vi "ATF - Datalog Redundant.vi"() -> ()   [LabVIEW 2022 SP3]
doc: "Datalog and display software modified"
uses:
  Source Code/Control/SeCrTs-Enum.ctl
  Source Code/Globals/SeCrTS-DD globals.vi
panel:
  out "Backlog Storage":i32
  out "Backlog Pump":i32
  out "Logging Mode":string
  out "cmd":bool=TRUE
  out "Storage Connected?":bool
  in  "Pump IP Address":string="169.254.31.109"
  in  "Storage IP Address":string="169.254.19.218"
  out "Datalog Title":string
  in  "Exit":bool
  out "Log Period(Min)":dbl
  out "Logging?":bool
  out "Pumb Connected?":bool
  out "error Out":errorcluster
  # "ATF PUMP AND STORAGE"
  # "DATALOG  REDUNDANT"
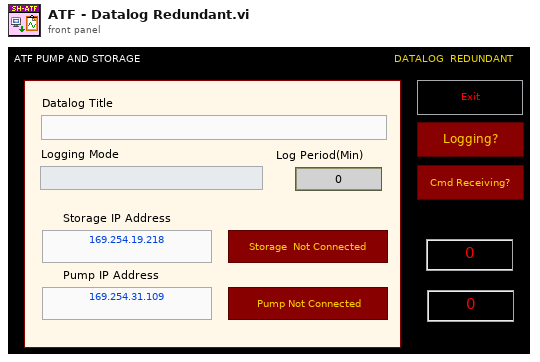
[diagram p1: front panel]
types:
  T1 = typedef "SeCrTs-Enum.ctl" = enum16{"Initialize", "Poll", "Establish ref", "Read", "Close", "Exit"}
  T2 = enum8{"Enabled", "Disabled", "Disabled and Grayed Out"}
  T3 = cluster{"C/NC":bool, "Start/Stop Log":bool[], "Log Name":string, "Config":cluster{"AO config":cluster{"Channel_Name":string, "Channel_Number":string, "Default_Value":dbl, "Units":string}[], "AI config":cluster{"Channel_Name":string, "Channel_Number":string, "Pre_Scale_min":dbl, "Pre_Scale_max":dbl, "Sensor_min":dbl, "Sensor_max":dbl, "Units":string}[], "DI config":cluster{"Channel_Name":string, "Channel_Number":string, "Default_Value":bool, "DI invert?":bool}[], "DO config":cluster{"Channel_Name":string, "Channel_Number":string, "Default_Value":bool, "DO invert?":bool}[], "TC config":cluster{"Channel_Name":string, "Channel_Number":string, "Pre_Scale_min":dbl, "Pre_Scale_max":dbl, "units":i32, " type":i32}[], "ACC config":cluster{"Channel_Name":string, "Channel_Number":string, "Pre_Scale_min":dbl, "Pre_Scale_max":dbl, "Terminal configuration":i32, "Sensitivity":dbl, "Sensitivity units":i32}[], "SG config":cluster{"Channel_Name":string, "Channel_Number":string, "Pre_Scale_min":dbl, "Pre_Scale_max":dbl}[], "Strain Gauge Settings":cluster{"poisson ratio":dbl, "nominal gage resistance":dbl, "gage factor":dbl}, "Bridge Settings":cluster{"voltage excitation value":dbl, "voltage excitation source":i32, "initial bridge voltage":dbl, "lead wire resistance":dbl, "strain configuration":i32}, "Sample Rate":cluster{"AI Sample Rate":dbl[], "AO Sample Rate":dbl[], "DI Sample Rate":dbl[], "TC Sample Rate":dbl[], "DO Sample Rate":dbl[], "SG Sample Rate":dbl[], "ACC Sample Rate":dbl[]}}, "Log min":dbl}
  T4 = cluster{"AO config":cluster{"Channel_Name":string, "Channel_Number":string, "Default_Value":dbl, "Units":string}[], "AI config":cluster{"Channel_Name":string, "Channel_Number":string, "Pre_Scale_min":dbl, "Pre_Scale_max":dbl, "Sensor_min":dbl, "Sensor_max":dbl, "Units":string}[], "DI config":cluster{"Channel_Name":string, "Channel_Number":string, "Default_Value":bool, "DI invert?":bool}[], "DO config":cluster{"Channel_Name":string, "Channel_Number":string, "Default_Value":bool, "DO invert?":bool}[], "TC config":cluster{"Channel_Name":string, "Channel_Number":string, "Pre_Scale_min":dbl, "Pre_Scale_max":dbl, "units":i32, " type":i32}[], "ACC config":cluster{"Channel_Name":string, "Channel_Number":string, "Pre_Scale_min":dbl, "Pre_Scale_max":dbl, "Terminal configuration":i32, "Sensitivity":dbl, "Sensitivity units":i32}[], "SG config":cluster{"Channel_Name":string, "Channel_Number":string, "Pre_Scale_min":dbl, "Pre_Scale_max":dbl}[], "Strain Gauge Settings":cluster{"poisson ratio":dbl, "nominal gage resistance":dbl, "gage factor":dbl}, "Bridge Settings":cluster{"voltage excitation value":dbl, "voltage excitation source":i32, "initial bridge voltage":dbl, "lead wire resistance":dbl, "strain configuration":i32}, "Sample Rate":cluster{"AI Sample Rate":dbl[], "AO Sample Rate":dbl[], "DI Sample Rate":dbl[], "TC Sample Rate":dbl[], "DO Sample Rate":dbl[], "SG Sample Rate":dbl[], "ACC Sample Rate":dbl[]}}
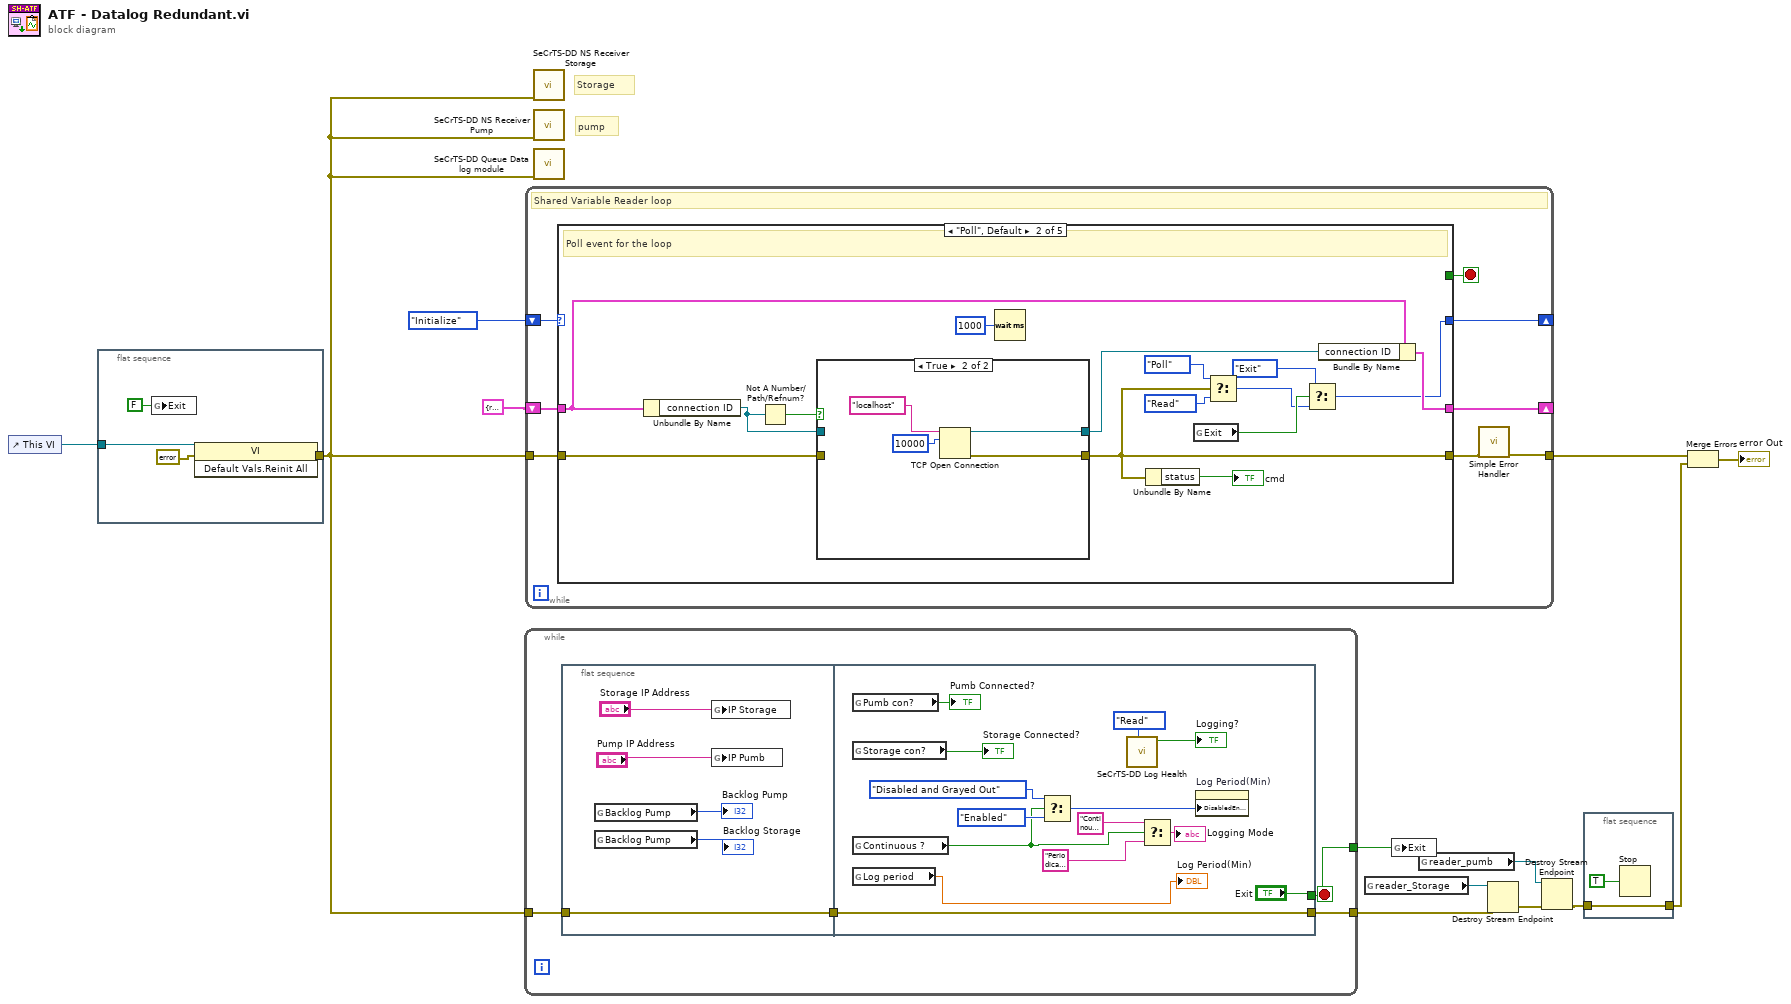
[diagram p0: block diagram]
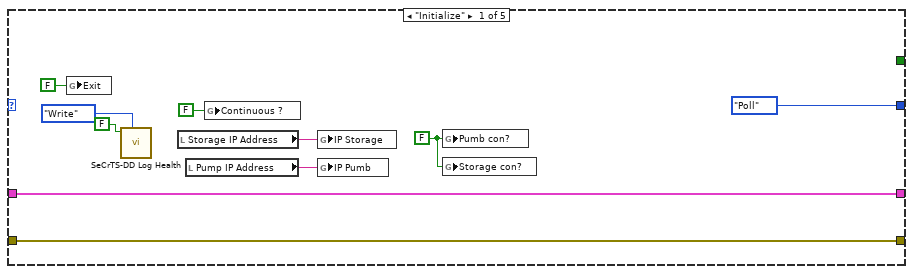
[diagram p2: hidden frame]
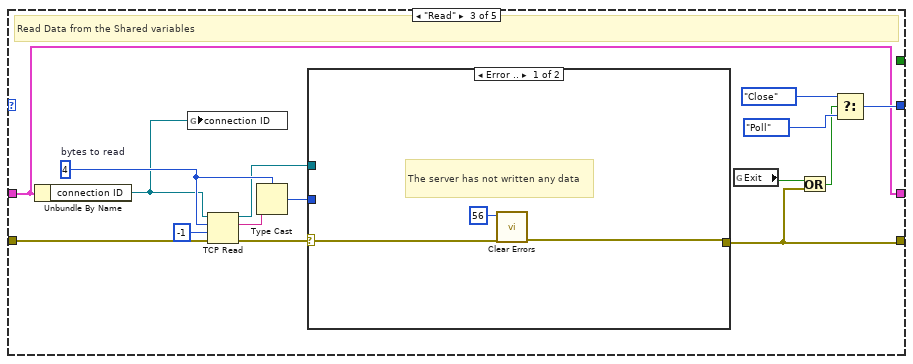
[diagram p4: hidden frame]
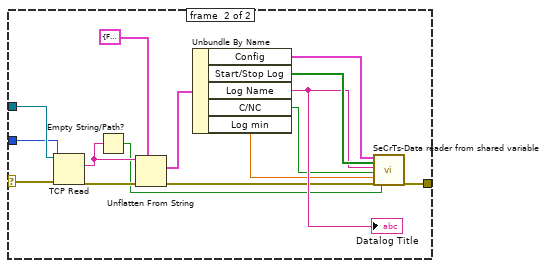
[diagram p5: hidden frame]
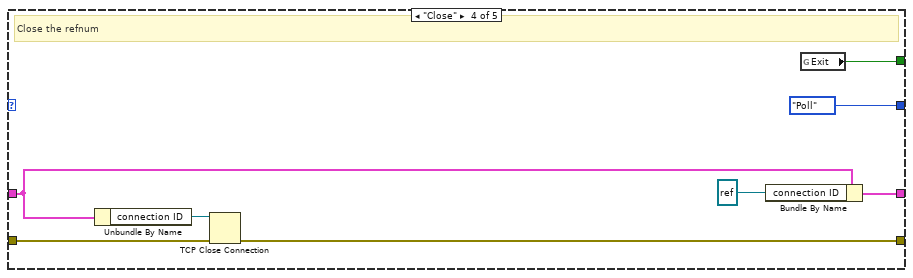
[diagram p6: hidden frame]
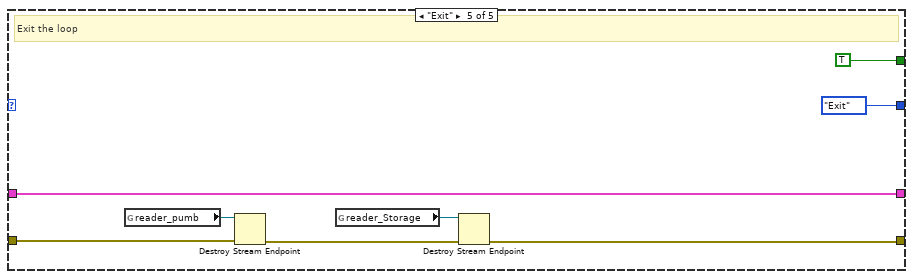
[diagram p7: hidden frame]
diagram:
  # "pump"
  # "Storage"
  n1 = control-ref of="This VI"() -> (w12:refnum<vi>)
  n2 = flat-sequence {
    tunnel: w12 -> [w17]
    tunnel: [w15] -> w1
    frame #0 {
      n3 = global write "SeCrTS-DD globals.vi" "Exit"(FALSE ("Exit")) -> ()
      n4 = invoke class="VI" method="Default Vals.Reinit All"(reference=w17, error in=errorcluster {"status"=FALSE, "code"=0, "source"=""}) -> (error out=w15:errorcluster)  [unwired: 1 in, 2 out]
    }
  }
  n5 = while {
    tunnel: w1 -> [w21]
    tunnel: [w19] -> w6
    tunnel: [w18] -> w9
    stop <- w18 stop-if-true
    n6 = flat-sequence {
      tunnel: w21 -> [w25]
      tunnel: [w25] -> w20
      tunnel: w20 -> [w33]
      tunnel: [w33] -> w19
      tunnel: ["Exit"] -> w18
      frame #0 {
        n7 = global read "SeCrTS-DD globals.vi" "Backlog Pump"() -> (→"Backlog Pump":i32)
        n8 = global read "SeCrTS-DD globals.vi" "Backlog Pump"() -> (→"Backlog Storage":i32)
        n9 = global write "SeCrTS-DD globals.vi" "IP Storage"("Storage IP Address") -> ()
        n10 = global write "SeCrTS-DD globals.vi" "IP Pumb"("Pump IP Address") -> ()
      }
      frame #1 {
        n11 = global read "SeCrTS-DD globals.vi" "Pumb con?"() -> (→"Pumb Connected?":bool)
        n12 = global read "SeCrTS-DD globals.vi" "Storage con?"() -> (→"Storage Connected?":bool)
        n13 = global read "SeCrTS-DD globals.vi" "Continuous ?"() -> (w30:bool)
        n14 = global read "SeCrTS-DD globals.vi" "Log period"() -> (→"Log Period(Min)":dbl)
        n15 = Select(t=T2."Disabled and Grayed Out" ("Disabled"), s=w30, f=T2."Enabled" ("Disabled")) -> (s? t:f=w39:T2)
        n16 = call "SeCrTS-DD Log Health.vi"("Enum"=enum16{"Read", "Write"}."Read") -> ("Log health R"=→"Logging?":bool)  [unwired: 9 in, 1 out]
        n17 = Select(t="Continous Logging Enabled" ("Logging Mode"), s=w30, f="Periodical Logging Enabled" ("Logging Mode")) -> (s? t:f=→"Logging Mode":string)
        n18 = property on="Log Period(Min)" class="DigNum (strict)"("DisabledEnum"=w39) -> ()  [unwired: 2 in, 2 out]
      }
    }
  }
  n19 = while {
    shift-right: [w46] -> _
    shift-left: SeCrTs-Enum."Initialize" -> [w48]
    shift-right: [w44] -> _
    shift-left: cluster{"connection ID":refnum<k5>} {"connection ID"=refnum} -> [w45]
    tunnel: w1 -> [w47]
    tunnel: [w41] -> w10
    stop <- w43 stop-if-true
    # "Shared Variable Reader loop"
    n20 = case shown="\"Poll\", Default" w48 {
      tunnel: w47 -> [w49 w67 w91 w118 w123]
      tunnel: [w49 w68 w82 w117 w121] -> w42
      tunnel: [SeCrTs-Enum."Poll" w60 w87 SeCrTs-Enum."Poll" SeCrTs-Enum."Exit"] -> w46
      tunnel: w45 -> [w57 w72 w86 w115 w126]
      tunnel: [w57 w73 w86 w116 w126] -> w44
      tunnel: [_ _ _ w113 TRUE] -> w43
      frame "Initialize" {
        w56 = FALSE ("Connect?")
        n21 = global write "SeCrTS-DD globals.vi" "Exit"(FALSE ("EXIT")) -> ()
        n22 = call "SeCrTS-DD Log Health.vi"("Enum"=enum16{"Read", "Write"}."Write", "Log health"=FALSE) -> ()  [unwired: 8 in, 2 out]
        n23 = local read "Storage IP Address"() -> (w55:string)
        n24 = local read "Pump IP Address"() -> (w51:string)
        n25 = global write "SeCrTS-DD globals.vi" "Continuous ?"(FALSE ("Continuous ?")) -> ()
        n26 = global write "SeCrTS-DD globals.vi" "IP Storage"(w55) -> ()
        n27 = global write "SeCrTS-DD globals.vi" "IP Pumb"(w51) -> ()
        n28 = global write "SeCrTS-DD globals.vi" "Pumb con?"(w56) -> ()
        n29 = global write "SeCrTS-DD globals.vi" "Storage con?"(w56) -> ()
      }
      frame "Poll", Default {
        # "Poll event for the loop"
        n30 = Unbundle By Name(w72) -> ("connection ID"=w70:refnum<k5>)
        n31 = Not A Number/Path/Refnum?(number/path/refnum=w70) -> (NaN/Path/Refnum?=w71:bool)
        n32 = case shown="True" w71 {
          tunnel: [w75 w76] -> w64
          tunnel: w70 -> [w75 _]
          tunnel: [w74 w79] -> w68
          tunnel: w67 -> [w74 _]
          frame False {
          }
          frame True {
            n33 = TCP Open Connection(address="localhost", remote port or service name=u16 10000) -> (connection ID=w76:refnum<k5>, error out=w79:errorcluster)  [unwired: 3 in]
          }
        }
        n34 = Wait (ms)(milliseconds to wait=u32 1000) -> ()  [unwired: 1 out]
        n35 = Unbundle By Name(w68) -> ("status"=→"cmd":bool)
        n36 = global read "SeCrTS-DD globals.vi" "Exit"() -> (w63:bool)
        n37 = Select(t=SeCrTs-Enum."Poll", s=w68, f=SeCrTs-Enum."Read") -> (s? t:f=w62:T1)
        n38 = Select(t=SeCrTs-Enum."Exit", s=w63, f=w62) -> (s? t:f=w60:T1)
        n39 = Bundle By Name(cluster=w72, "connection ID"=w64) -> (w73:cluster{"connection ID":refnum<k5>})
      }
      frame "Read" {
        w93 = 4  # bytes to read
        # "Read Data from the Shared variables"
        n40 = Unbundle By Name(w86) -> ("connection ID"=w80:refnum<k5>)
        n41 = global write "SeCrTS-DD globals.vi" "connection ID"(w80) -> ()
        n42 = TCP Read(connection ID=w80, bytes to read=w93, error in (no error)=w91, 9:-1 ("timeout ms (25000)")) -> (connection ID out=w90:refnum<k5>, data out=w94:string, error out=w85:errorcluster)  [unwired: 1 in]
        n43 = Type Cast(type=w93, x=w94) -> (*(type *) &x=w92:i32)
        n44 = case shown="Error .." w85 {
          selector: w85 -> [w97 w111]
          tunnel: w90 -> [_ w112]
          tunnel: [w96 w98] -> w82
          tunnel: w92 -> [_ w110]
          frame #0 {
            # "The server has not written any data"
            n45 = call <vilib>:"Clear Errors.vi"("error in (no error)"=w97, "specific error code to clear (0: all)"=56) -> ("error out"=w96:errorcluster)  [unwired: 4 in, 1 out]
          }
          frame #1 {
            n46 = TCP Read(connection ID=w112, bytes to read=w110, error in (no error)=w111) -> (data out=w102:string, error out=w101:errorcluster)  [unwired: 2 in, 1 out]
            n47 = Empty String/Path?(string/path=w102) -> (empty?=w100:bool)
            n48 = Unflatten From String(type=T3 {"C/NC"=FALSE, "Start/Stop Log"=[], "Log Name"="", "Config"={"AO config"=[], "AI config"=[], "DI config"=[], "DO config"=[], "TC config"=[], "ACC config"=[], "SG config"=[], "Strain Gauge Settings"={"poisson ratio"=0.0, "nominal gage resistance"=0.0, "gage factor"=0.0}, "Bridge Settings"={"voltage excitation value"=0.0, "voltage excitation source"=0, "initial bridge voltage"=0.0, "lead wire resistance"=0.0, "strain configuration"=0}, "Sample Rate"={"AI Sample Rate"=[], "AO Sample Rate"=[], "DI Sample Rate"=[], "TC Sample Rate"=[], "DO Sample Rate"=[], "SG Sample Rate"=[], "ACC Sample Rate"=[]}}, "Log min"=0.0} ("Cluster"), binary string=w102, error in (no error)=w101) -> (value=w108:T3, error out=w99:errorcluster)  [unwired: 2 in, 1 out]
            n49 = Unbundle By Name(w108) -> ("Config"=w107:T4, "Start/Stop Log"=w106:bool[], "Log Name"=w105:string, "C/NC"=w104:bool, "Log min"=w103:dbl)
            "Datalog Title" <- w105
            n50 = call "SeCrTs-Data reader from shared variable.vi"("Config"=w107, "Start/Stop Log"=w106, "Log Name"=w105, "C/NC"=w104, "Log min"=w103, "error IO"=w99, "empty?"=w100) -> ("error out"=w98:errorcluster)  [unwired: 12 in]
          }
        }
        n51 = global read "SeCrTS-DD globals.vi" "Exit"() -> (w83:bool)
        n52 = Or(x=w83, y=w82) -> (x .or. y?=w81:bool)
        n53 = Select(t=SeCrTs-Enum."Close", s=w81, f=SeCrTs-Enum."Poll") -> (s? t:f=w87:T1)
      }
      frame "Close" {
        # "Close the refnum"
        n54 = Unbundle By Name(w115) -> ("connection ID"=w119:refnum<k5>)
        n55 = TCP Close Connection(connection ID=w119, error in (no error)=w118) -> (error out=w117:errorcluster)  [unwired: 1 in, 1 out]
        n56 = Bundle By Name(cluster=w115, "connection ID"=refnum<k5> refnum) -> (w116:cluster{"connection ID":refnum<k5>})
        n57 = global read "SeCrTS-DD globals.vi" "Exit"() -> (w113:bool)
      }
      frame "Exit" {
        # "Exit the loop"
        n58 = global read "SeCrTS-DD globals.vi" "reader_pumb"() -> (w125:refnum<k21>)
        n59 = Destroy Stream Endpoint(8:w123, 11:w125) -> (0:w122:errorcluster)
        n60 = global read "SeCrTS-DD globals.vi" "reader_Storage"() -> (w124:refnum<k21>)
        n61 = Destroy Stream Endpoint(8:w122, 11:w124) -> (0:w121:errorcluster)
      }
    }
    n62 = call <vilib>:"Simple Error Handler.vi"("error in (no error)"=w42) -> ("error out"=w41:errorcluster)  [unwired: 4 in, 4 out]
  }
  n63 = call "SeCrTS-DD NS Receiver Storage.vi"("error in"=w1) -> ()  [unwired: 11 in]
  n64 = call "SeCrTS-DD NS Receiver Pump.vi"("error in"=w1) -> ()  [unwired: 11 in]
  n65 = call "SeCrTS-DD Queue Data log module.vi"("error in"=w1) -> ()  [unwired: 10 in, 1 out]
  n66 = global read "SeCrTS-DD globals.vi" "reader_Storage"() -> (w7:refnum<k21>)
  n67 = global write "SeCrTS-DD globals.vi" "Exit"(w9) -> ()
  n68 = global read "SeCrTS-DD globals.vi" "reader_pumb"() -> (w8:refnum<k21>)
  n69 = Destroy Stream Endpoint(8:w6, 11:w7) -> (0:w5:errorcluster)
  n70 = Destroy Stream Endpoint(8:w5, 11:w8) -> (0:w3:errorcluster)
  n71 = flat-sequence {
    tunnel: w3 -> [w130]
    tunnel: [w130] -> w2
    frame #0 {
      n72 = Stop(stop? (T)=TRUE) -> ()
    }
  }
  n73 = Merge Errors(w10, w2) -> (→"error Out":errorcluster)
